vi "phan_upgrade13_2.vi"() -> ()   [LabVIEW 2019]
uses:
  <vilib>/Analysis/Matrix/Datatypes/RealMatrix.ctl
  <vilib>/Platform/TimedLoop/XDataNode/timing_clust.ctl
  <vilib>/Platform/TimedLoop/XDataNode/nitl_modes.ctl
  <vilib>/Platform/TimedLoop/XDataNode/wakeup.ctl
  <vilib>/imath/engines/lvmath2/RunTimeEngine/IndexRead/NIMS V(S).vi
  <instcachedir>/0/NIMS V(S)_0488751826AF41519A22953C041130DC.lvgen/NIMS V(S)_0488751826AF41519A22953C041130DC_000.vi
  <vilib>/imathl/engines/lvmath/Functions/Error Handling/Create Error.vi
  <vilib>/imath/engines/lvmath2/RunTimeEngine/NodeEndStatement/NIMS_NodeEndStatement_Output.vi
  <instcachedir>/0/NIMS_NodeEndStatement_Output_53EC0D466D134D7ABD903AC30B43404B.lvgen/NIMS_NodeEndStatement_Output_53EC0D466D134D7ABD903AC30B43404B_001.vi
  <vilib>/imath/engines/lvmath2/RunTimeEngine/ErrorHandling/NIMS_Finalize Error.vi
  <vilib>/imath/engines/lvmath2/RunTimeEngine/ArithmeticOperatorToken/NIMS_ArithmeticOperator_multmx(M,CV)-internal.vi
  <instcachedir>/0/NIMS_ArithmeticOperator_multmx(M,CV)-internal_2C55777844884EEDB828A940D397C7D0.lvgen/NIMS_ArithmeticOperator_multmx(M,CV)-internal_2C55777844884EEDB828A940D397C7D0_001.vi
  <vilib>/Analysis/Matrix/Numeric/Conversions/Matrix To Array - RM.vi
  <vilib>/imath/engines/lvmath2/RunTimeEngine/BuiltInFunctions/is_empty/NIMS_is_empty(GM).vi
  <instcachedir>/0/NIMS_is_empty(GM)_AF8F13F4B7FD436CB1855477E2504B8A.lvgen/NIMS_is_empty(GM)_AF8F13F4B7FD436CB1855477E2504B8A_004.vi
  <vilib>/imath/engines/lvmath2/RunTimeEngine/ArithmeticOperatorToken/NIMS_ArithmeticOperator_minus.vi
  <instcachedir>/0/NIMS_ArithmeticOperator_minus_12BFF9710EA5430A9EE87C5BC3F65186.lvgen/NIMS_ArithmeticOperator_minus_12BFF9710EA5430A9EE87C5BC3F65186_002.vi
  <vilib>/imath/engines/lvmath2/RunTimeEngine/ArithmeticOperatorToken/NIMS_ArithmeticOperator_plus.vi
  <instcachedir>/0/NIMS_ArithmeticOperator_plus_5C9385B0197D46E2B844C41E02F9EC39.lvgen/NIMS_ArithmeticOperator_plus_5C9385B0197D46E2B844C41E02F9EC39_003.vi
  <vilib>/imath/engines/lvmath2/RunTimeEngine/ErrorHandling/NIMS_Create Error From Enums.vi
  <vilib>/imath/engines/lvmath2/RunTimeEngine/RowToken/NIMS_RowToken_M_M.vi
  <instcachedir>/0/NIMS_RowToken_M_M_21FE36D058524603B8B587AC30FD72C2.lvgen/NIMS_RowToken_M_M_21FE36D058524603B8B587AC30FD72C2_004.vi
  <vilib>/imath/engines/lvmath2/RunTimeEngine/ArithmeticOperatorToken/NIMS_ArithmeticOperator_multmx(M,CV).vi
  <instcachedir>/0/NIMS_ArithmeticOperator_multmx(M,CV)_1D61EED49E1847F3B05DBB8EDD2FBF8F.lvgen/NIMS_ArithmeticOperator_multmx(M,CV)_1D61EED49E1847F3B05DBB8EDD2FBF8F_000.vi
  <vilib>/imath/engines/lvmath2/RunTimeEngine/IndexRead/NIMS M(S).vi
  <instcachedir>/0/NIMS M(S)_B826C018497E4940AE96BD27B540B6FB.lvgen/NIMS M(S)_B826C018497E4940AE96BD27B540B6FB_000.vi
  <vilib>/imath/engines/lvmath2/RunTimeEngine/BuiltInFunctions/abs/NIMS_abs(signed).vi
  <instcachedir>/0/NIMS_abs(signed)_C4FCB8E6058B49B797C7C8D53CA5F6EC.lvgen/NIMS_abs(signed)_C4FCB8E6058B49B797C7C8D53CA5F6EC_000.vi
  <vilib>/imath/engines/lvmath2/RunTimeEngine/VariableToken/NIMS_VariableToken_CondDefined.vi
  <instcachedir>/0/NIMS_VariableToken_CondDefined_30C3C94EAC01413DA882E848DEC89944.lvgen/NIMS_VariableToken_CondDefined_30C3C94EAC01413DA882E848DEC89944_003.vi
  <instcachedir>/0/NIMS_VariableToken_CondDefined_30C3C94EAC01413DA882E848DEC89944.lvgen/NIMS_VariableToken_CondDefined_30C3C94EAC01413DA882E848DEC89944_004.vi
  <instcachedir>/0/NIMS_VariableToken_CondDefined_30C3C94EAC01413DA882E848DEC89944.lvgen/NIMS_VariableToken_CondDefined_30C3C94EAC01413DA882E848DEC89944_001.vi
  <vilib>/Analysis/Matrix/Numeric/Conversions/Array To Matrix - RA2.vi
  <instcachedir>/0/NIMS_VariableToken_CondDefined_30C3C94EAC01413DA882E848DEC89944.lvgen/NIMS_VariableToken_CondDefined_30C3C94EAC01413DA882E848DEC89944_005.vi
  <vilib>/imath/engines/lvmath/Functions/Error Handling/MergeErrorsWrapper.vi
  <instcachedir>/0/NIMS_NodeEndStatement_Output_53EC0D466D134D7ABD903AC30B43404B.lvgen/NIMS_NodeEndStatement_Output_53EC0D466D134D7ABD903AC30B43404B_012.vi
  <instcachedir>/0/NIMS_NodeEndStatement_Output_53EC0D466D134D7ABD903AC30B43404B.lvgen/NIMS_NodeEndStatement_Output_53EC0D466D134D7ABD903AC30B43404B_010.vi
  <vilib>/platform/TimedLoop/XDataNode/XDataNode.xnode
  <vilib>/Platform/TimedLoop/XDataNode/XDNodeRunTimeDep.lvlib
  <vilib>/ptbypt/NI_PtbyPt.lvlib
  <vilib>/Analysis/Matrix/NI_Matrix.lvlib
panel:
  in  "yA":dbl
  in  "xA":dbl
  out "data out":string
  out "sosanh":dbl
  out "error out 2":errorcluster
  out "phi_k":dbl
  out "y_k":dbl
  out "x_k":dbl
  out "Real Matrix 2":T1
  out "Real Matrix":T1
  out "e_k":T1 caption="Real Matrix"
  out "error out":errorcluster
  out "y":dbl(graph)
  out "x":dbl(graph)
  out "y_1":dbl
  out "x_1":dbl
  out "y_0":dbl
  out "x_0":dbl
  out "wpre":dbl
  out "yo":dbl
  out "xo":dbl
  out "phi_ph":dbl
  out "wdk":dbl
  out "phi_sp":dbl
  in  "Kiw":dbl
  in  "Kpw":dbl=3.0
  in  "Kdw":dbl
  out "Vxdk":dbl
  out "Vydk":dbl
  out "Ts":dbl=10.0
  out "sailechvitri":cluster{"e_phi":dbl, "e_x":dbl, "e_y":dbl}(graph)
  in  "Kdxy":dbl
  in  "Kixy":dbl
  in  "Kpxy":dbl=4.0
  in  "?":T2(tab)
  out "time":dbl
  in  "phi_start":dbl=1.57 format="%#_13g"
  in  "phi_end":dbl=18.85
  in  "x0":dbl
  in  "w":dbl=0.2
  in  "y0":dbl
  in  "R":dbl=1.0
  in  "R":dbl=0.6
  in  "phi_end":dbl=18.85
  in  "phi_start":dbl format="%#_13g"
  in  "x0":dbl
  in  "w":dbl=0.5
  out "time 2":dbl
  in  "y0":dbl
  out "time":dbl
  in  "x":dbl
  in  "y":dbl
  in  "CONT":bool
  in  "vantoc":dbl=0.3
  in  "T":dbl
  out "time":dbl
  in  "camera update":bool
  out "xd":dbl
  out "yd":dbl
  out "phi":dbl
  out "time 3":dbl
  in  "phi_start 2":dbl format="%#_13g"
  in  "phi_end 2":dbl=31.4
  in  "x0 2":dbl
  in  "w 2":dbl=0.2
  in  "y0 2":dbl
  out "w_ph3":dbl
  out "w_ph2":dbl
  out "w_ph1":dbl
  in  "RESETMAP":bool=TRUE caption="Reset"
  out "duty3":dbl
  out "duty2":dbl
  out "duty1":dbl
  in  "RESET":bool
  out "Y_sp":dbl
  out "X_sp":dbl
  out "Y_ph":dbl
  out "X_ph":dbl
  out "Map":cluster{"Y":dbl[], "Y":dbl[]}[](graph)
  out "V3_sp":dbl
  out "V3_ph":dbl
  out "VAN TOC":T3(graph)
  in  "Kdv":dbl
  in  "Kiv":dbl=52.63
  in  "Kpv":dbl=1.337
  out "V2_ph":dbl
  out "V1_ph":dbl
  out "V2_sp":dbl
  out "V1_sp":dbl
  in  "START":bool
  # "HE THONG"
  # "PID VI TRI"
  # "PID TOC DO"
  # "VI TRI DIEU KHIEN\n(m)"
  # "VI TRI PHAN HOI\n(m)"
  # "Van toc dat"
  # "VAN TOC DIEU KHIEN\n(m/s)"
  # "VAN TOC PHAN HOI\n(m/s)"
  # "DUTY"
  # "TOC DO PHAN HOI (rad/s)"
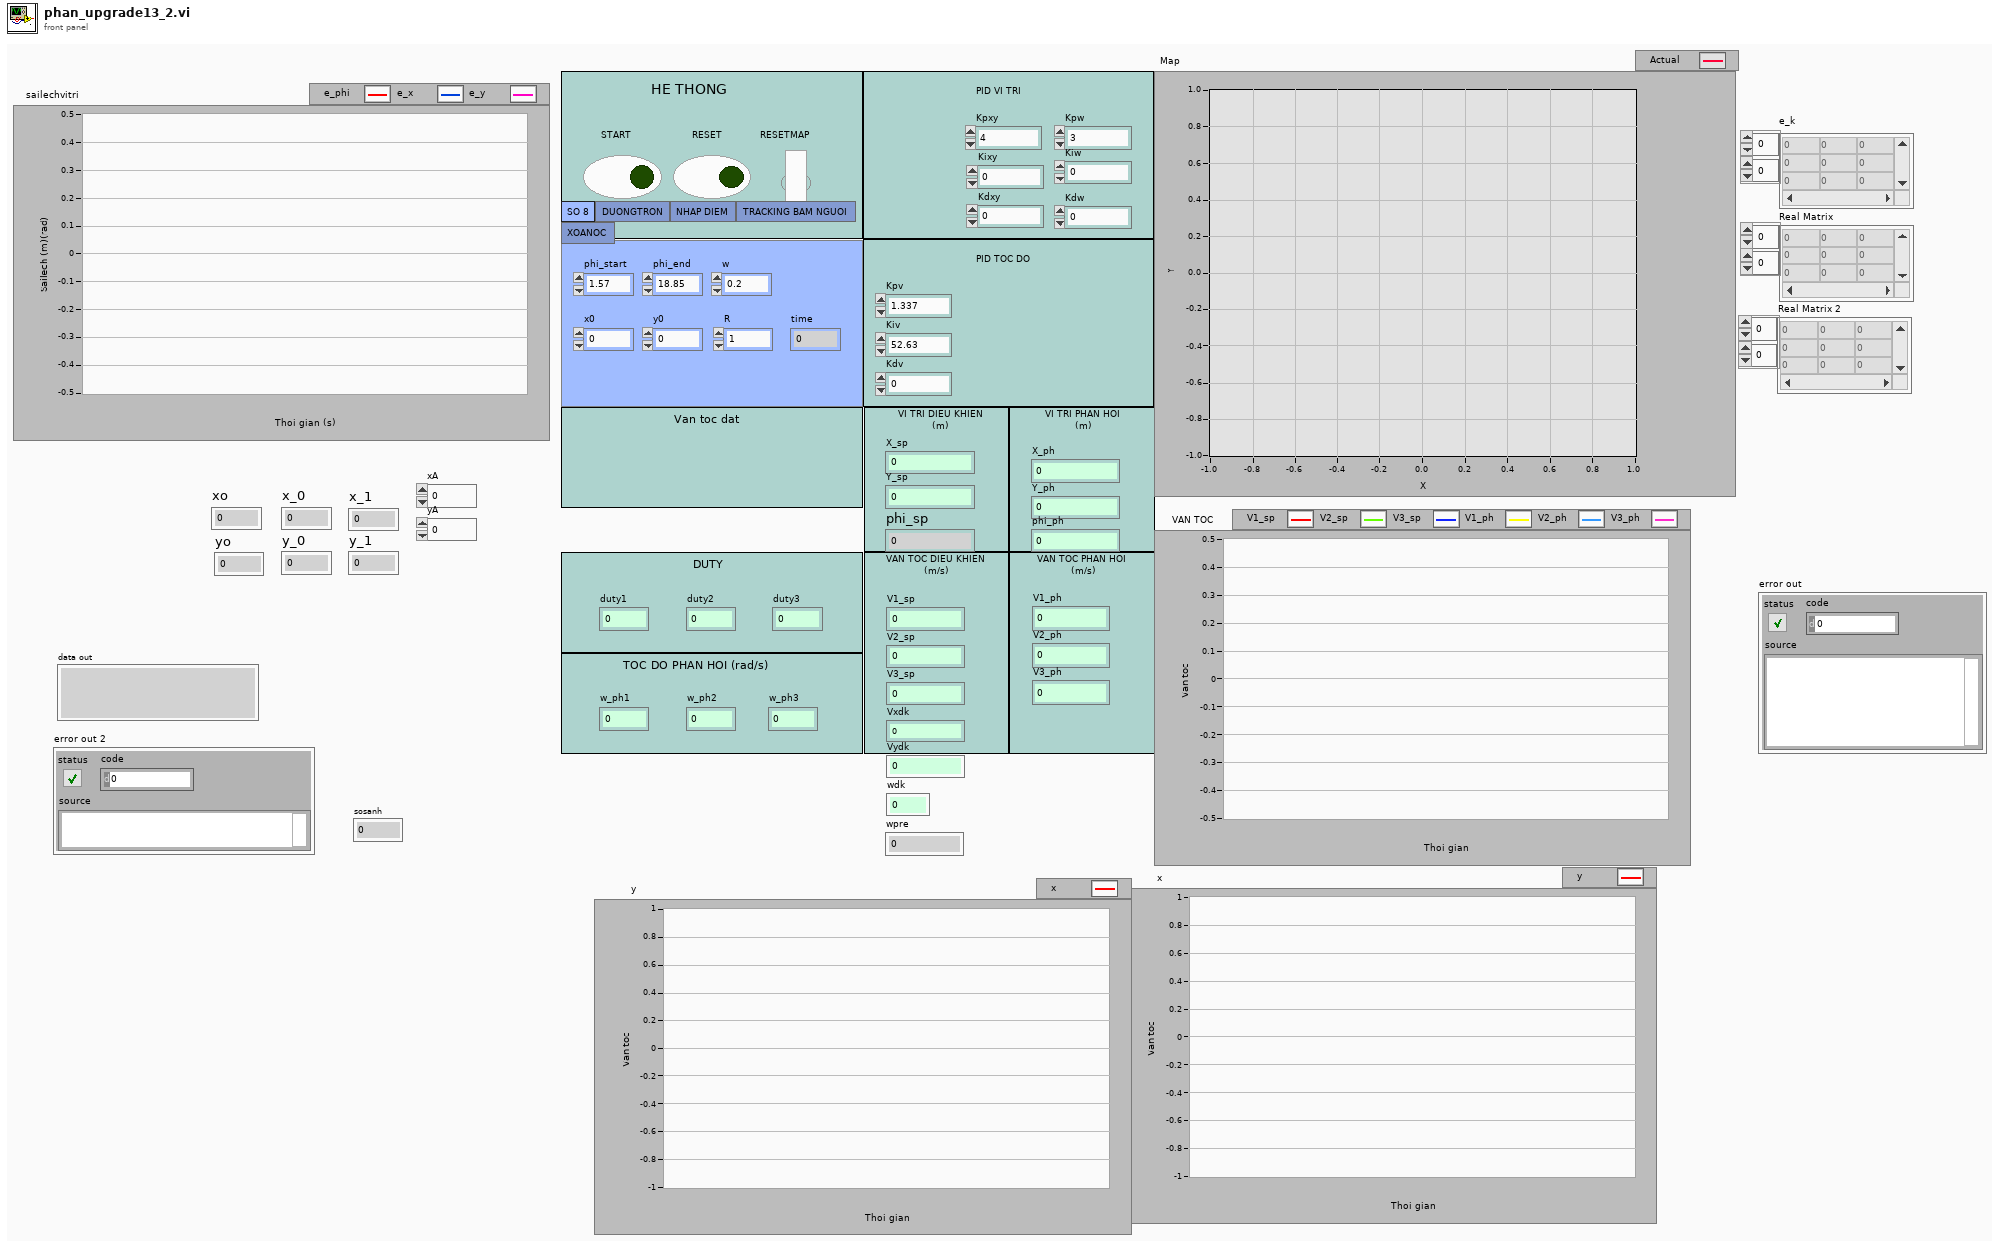
[diagram p1: front panel]
types:
  T1 = typedef "NI_Matrix.lvlib/RealMatrix.ctl" = dbl[][]
  T2 = enum32{"SO 8", "DUONGTRON", "NHAP DIEM", "TRACKING BAM NGUOI", "XOANOC"}
  T3 = cluster{dbl, dbl, "V1_ph":dbl, "V2_ph":dbl, dbl, "V3_ph":dbl}
  T4 = typedef "XDNodeRunTimeDep.lvlib/timing_clust.ctl" = cluster{"Expected End [f-1]":u64, "Actual End [f-1]":u64, "Finished Late? [f-1]":bool, "Expected End [i-1]":u64, "Actual End [i-1]":u64, "Finished Late? [i-1]":bool, "Expected Start [i]":u64, "Actual Start [i]":u64, "Expected Start [f]":u64, "Actual Start [f]":u64, "Source Name":string, "Structure Name":string, "Period":i64, "Deadline":i64, "Offset":i64, "Start":i64, "Priority":i32, "Timeout":i32, "Mode":T5, "Wakeup Reason":T6, "Error":errorcluster, "Source Type":string, "Secondary Source Type":string, "Global End Time":u64, "Global Start Time":u64, "Frame Duration":u64, "Iteration Duration":u64, "Assigned CPU":i32, "I/O Scan Engine Mode":u32}
  T5 = typedef "XDNodeRunTimeDep.lvlib/nitl_modes.ctl" = enum32{"No Change", "Process missed periods, maintain original phase", "Discard missed periods, maintain original phase", "Process missed periods, ignore original phase", "Discard missed periods, ignore original phase"}
  T6 = typedef "XDNodeRunTimeDep.lvlib/wakeup.ctl" = enum32{"Normal", "Aborted", "Asynchronous wakeup", "Timing source error", "Timed loop error", "Timeout"}
  T7 = enum16{"Standard", "Buffered", "CRLF", "Immediate"}
  T8 = cluster{"V1_sp":dbl, "V2_sp":dbl, "V3_sp":dbl, "V_ph1":dbl, "V_ph2":dbl, "V_ph3":dbl}
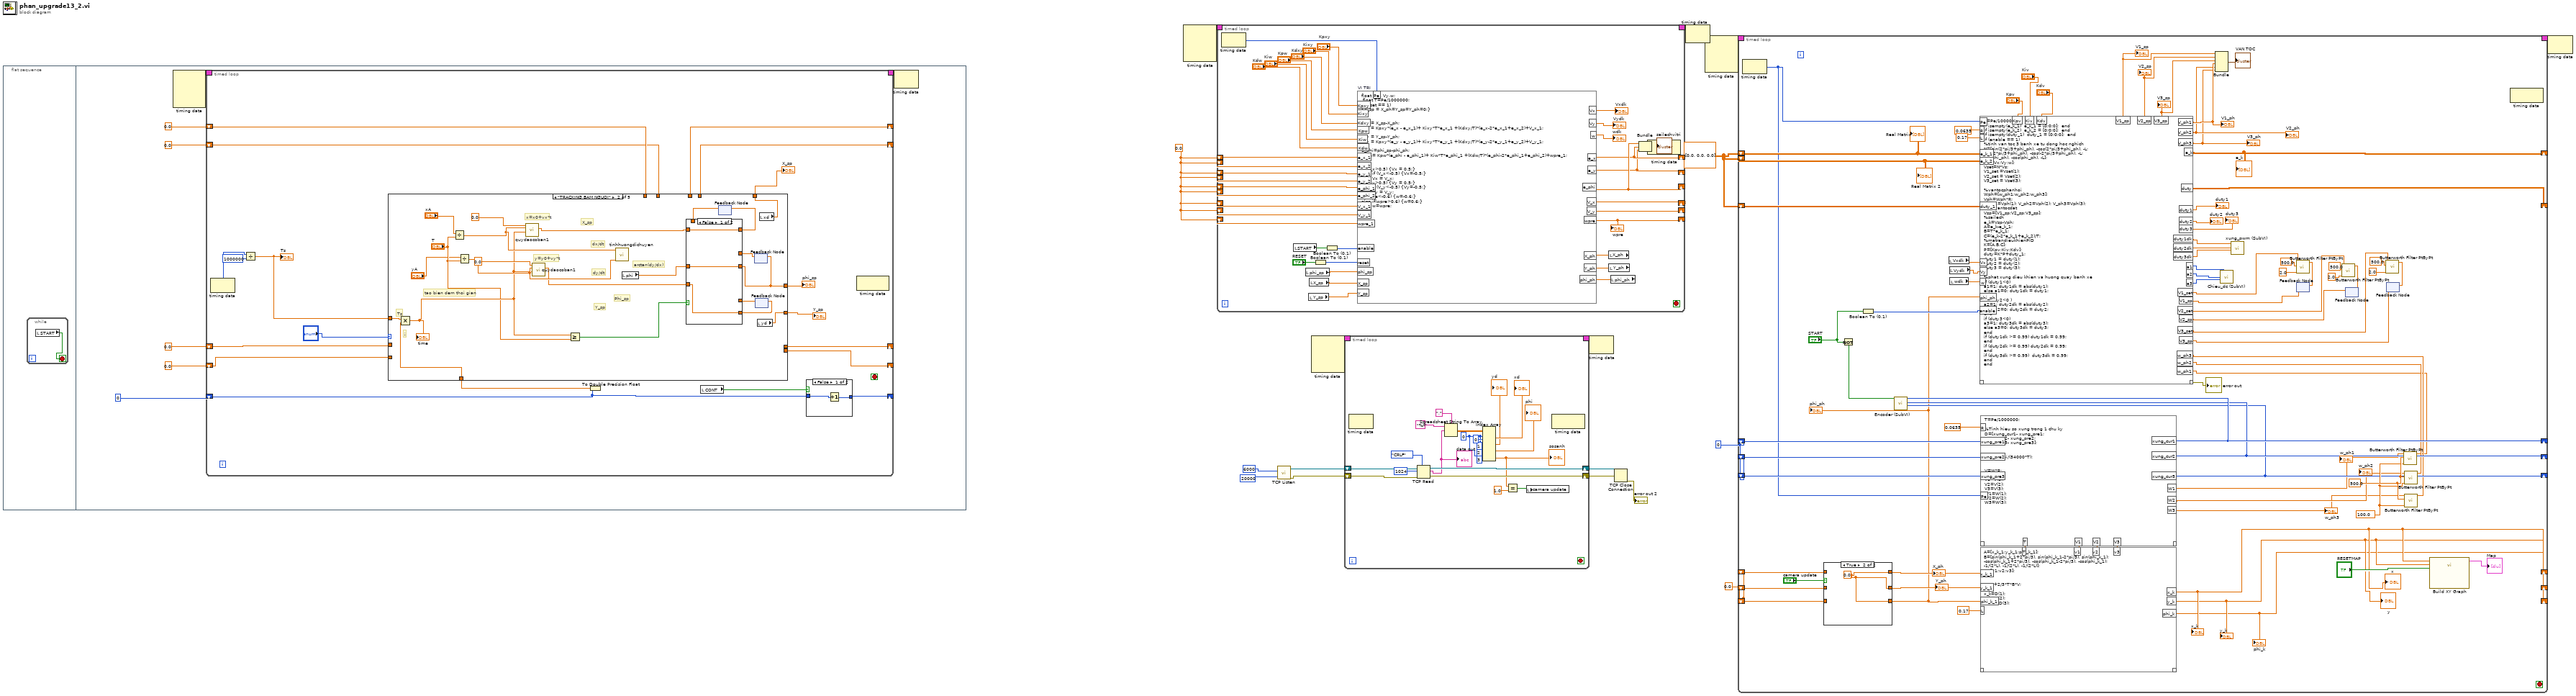
[diagram p0: block diagram]
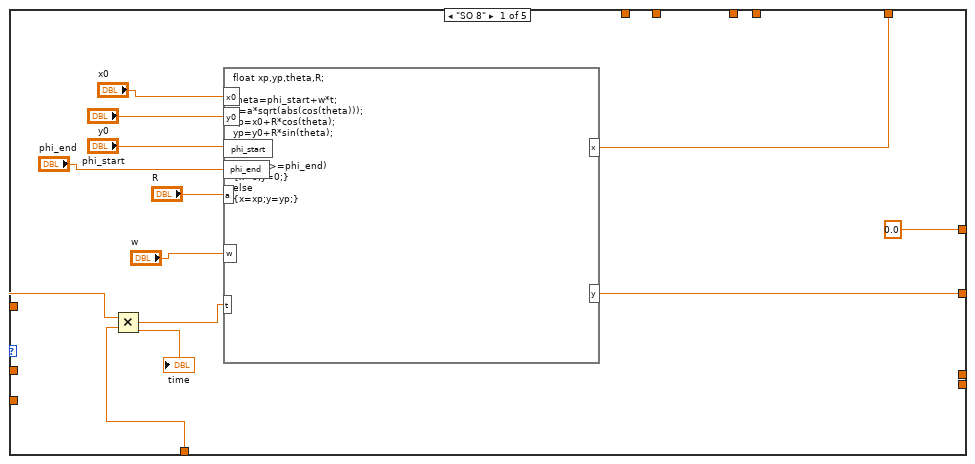
[diagram p2: hidden frame]
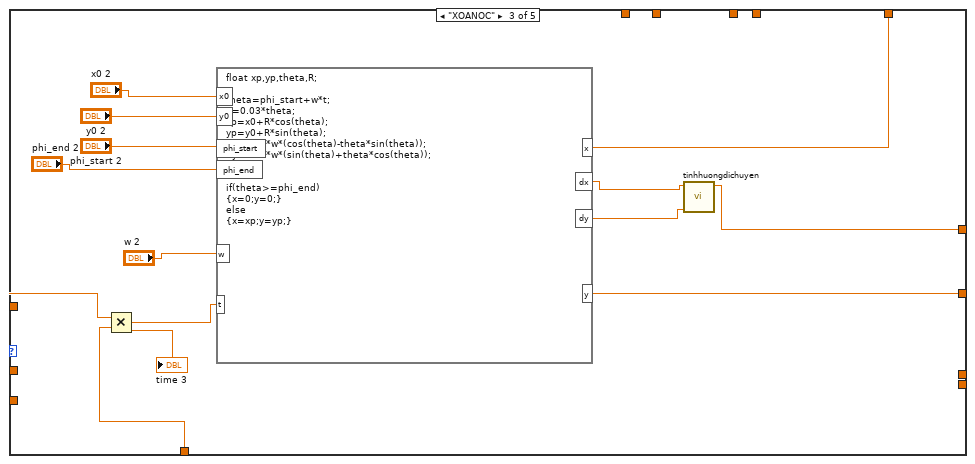
[diagram p4: hidden frame]
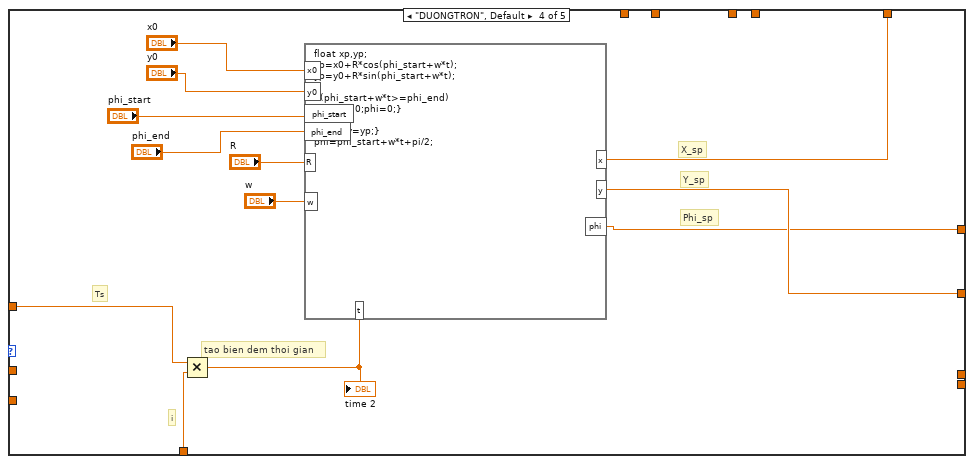
[diagram p5: hidden frame]
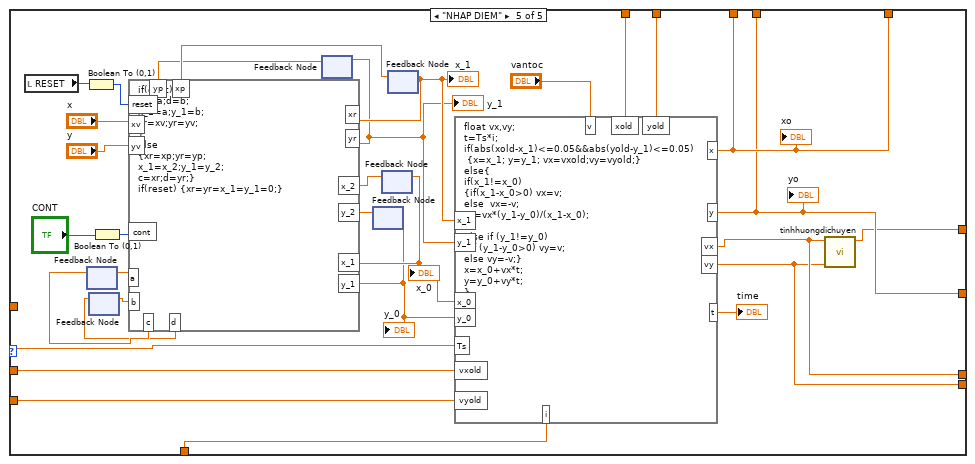
[diagram p6: hidden frame]
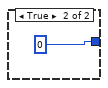
[diagram p7: hidden frame]
diagram:
  w11 = T1 [[0.0], [0.0], [0.0]] ("Real Matrix")
  w12 = 0 ("Counter Value")
  w13 = 0.0 ("e_x")
  w10 = 0.0 ("e1")
  n1 = flat-sequence {
    frame #0 {
      n2 = while {
        stop <- w18 stop-if-true
        n3 = local read "START"() -> (w18:bool)
      }
    }
    frame #1 {
      n4 = node-c288() -> (w25:T4)  [unwired: 4 in]
      n5 = timed-loop {
        timing: w25 -> [_]
        timing-out: [_] -> w24
        shift-right: [w43] -> _
        shift-left: 0 -> [w42]
        shift-right: [w34] -> _
        shift-left: 0.0 -> [w32]
        shift-right: [w33] -> _
        shift-left: 0.0 -> [w31]
        shift-right: [w30] -> _
        shift-left: 0.0 ("x") -> [w28]
        shift-right: [w29] -> _
        shift-left: 0.0 ("y") -> [w27]
        stop <- _ stop-if-true
        n6 = node-c288() -> (w41:i64)  [unwired: 1 in]
        n7 = Divide(x=w41, y=i64 1000000) -> (x/y=w39:dbl)
        "Ts" <- w39
        n8 = To Double Precision Float(number=w42) -> (double precision float=w44:dbl)
        n9 = case shown="\"TRACKING BAM NGUOI\"" "?" {
          tunnel: w44 -> [w55 w78 w90 w108 w140]
          tunnel: [w47 w58 w88 w100 w114] -> w38
          tunnel: [w46 w57 w89 w99 w113] -> w37
          tunnel: [0.0 ("phi_0") w65 w85 w98 w110] -> w36
          tunnel: w39 -> [w56 w77 w91 w109 w120]
          tunnel: [_ _ _ _ w118] -> w34
          tunnel: [_ _ _ _ w117] -> w33
          tunnel: w32 -> [_ _ _ _ w116]
          tunnel: w31 -> [_ _ _ _ w115]
          tunnel: [_ _ _ _ w114] -> w30
          tunnel: [_ _ _ _ w113] -> w29
          tunnel: w28 -> [_ _ _ _ w112]
          tunnel: w27 -> [_ _ _ _ w111]
          frame "SO 8" {
            n10 = Multiply(x=w56, y=w55) -> (x*y=w54:dbl)
            "time" <- w54
            n11 = formula code="float xp,yp,theta,R;\n\ntheta=phi_start+w*t;\nR=a*sqrt(abs(cos(theta)));\nxp=x0+R*cos(theta);\nyp=y0+R*sin(theta);\n\n\nif(theta>=phi_end)\n{x=0;y=0;}\nelse\n{x=xp;y=yp;}"("t"=w54, "w"="w", "x0"="x0", "y0"="y0", "phi_start"="phi_start", "phi_end"="phi_end", "a"="R") -> ("x"=w47:dbl, "y"=w46:dbl)
          }
          frame "TRACKING BAM NGUOI" {
            # "Y_sp"
            # "Phi_sp"
            # "X_sp"
            # "arctan(dy/dx)"
            # "dy/dt"
            # "dx/dt"
            # "Ts"
            # "i"
            # "y=y0+vy*t"
            # "x=x0+vx*t"
            # "tao bien dem thoi gian"
            n12 = Multiply(x=w77, y=w78) -> (x*y=w72:dbl)
            "time" <- w72
            n13 = Divide(x="xA", y="T") -> (x/y=w74:dbl)
            n14 = Divide(x="yA", y="T") -> (x/y=w73:dbl)
            n15 = call "quydaocoban1.vi"("t"=w72, "v"=w74, "S0"=0.0 ("x0")) -> ("S"=w69:dbl)  [unwired: 8 in]
            n16 = call "quydaocoban1.vi"("t"=w72, "v"=w73, "S0"=0.0 ("y0")) -> ("S"=w68:dbl)  [unwired: 8 in]
            n17 = Greater Or Equal?(x=w72, y="T") -> (x >= y?=w70:bool)
            n18 = call "tinhhuongdichuyen.vi"("dy"=w73, "dx"=w74) -> ()  [unwired: 9 in, 1 out]
            n19 = local read "phi"() -> (w61:dbl)
            n20 = feedback #1() -> (w66:dbl)  [unwired: 1 in]
            n21 = feedback #2() -> (w64:dbl)  [unwired: 1 in]
            n22 = feedback #3() -> (w62:dbl)  [unwired: 1 in]
            n23 = case shown="False" w70 {
              tunnel: w69 -> [w81 _]
              tunnel: [w81 w84] -> w67
              tunnel: w61 -> [w80 _]
              tunnel: [w80 w83] -> w65
              tunnel: w68 -> [w79 _]
              tunnel: [w79 w82] -> w63
              tunnel: w66 -> [_ w84]
              tunnel: w64 -> [_ w83]
              tunnel: w62 -> [_ w82]
              frame False {
              }
              frame True {
              }
            }
            n24 = feedback-in #1(w67) -> ()
            n25 = feedback-in #2(w65) -> ()
            n26 = feedback-in #3(w63) -> ()
            n27 = local read "yd"() -> (w57:dbl)
            n28 = local read "xd"() -> (w58:dbl)
          }
          frame "XOANOC" {
            n29 = Multiply(x=w91, y=w90) -> (x*y=w97:dbl)
            "time 3" <- w97
            n30 = formula code="float xp,yp,theta,R;\n\ntheta=phi_start+w*t;\nR=0.03*theta;\nxp=x0+R*cos(theta);\nyp=y0+R*sin(theta);\ndx=0.03*w*(cos(theta)-theta*sin(theta));\ndy=0.03*w*(sin(theta)+theta*cos(theta));\n\n\nif(theta>=phi_end)\n{x=0;y=0;}\nelse\n{x=xp;y=yp;}"("t"=w97, "w"="w 2", "x0"="x0 2", "y0"="y0 2", "phi_start"="phi_start 2", "phi_end"="phi_end 2") -> ("x"=w88:dbl, "y"=w89:dbl, "dx"=w87:dbl, "dy"=w86:dbl)
            n31 = call "tinhhuongdichuyen.vi"("dy"=w86, "dx"=w87) -> ("phi"=w85:dbl)  [unwired: 9 in]
          }
          frame "DUONGTRON", Default {
            # "Phi_sp"
            # "Y_sp"
            # "X_sp"
            # "i"
            # "Ts"
            # "tao bien dem thoi gian"
            n32 = Multiply(x=w109, y=w108) -> (x*y=w107:dbl)
            "time 2" <- w107
            n33 = formula code="float xp,yp;\nxp=x0+R*cos(phi_start+w*t);\nyp=y0+R*sin(phi_start+w*t);\n\nif(phi_start+w*t>=phi_end)\n{x=0;y=0;phi=0;}\nelse\n{x=xp;y=yp;}\nphi=phi_start+w*t+pi/2;"("t"=w107, "w"="w", "x0"="x0", "y0"="y0", "phi_start"="phi_start", "phi_end"="phi_end", "R"="R") -> ("x"=w100:dbl, "y"=w99:dbl, "phi"=w98:dbl)
          }
          frame "NHAP DIEM" {
            n34 = local read "RESET"() -> (w122:bool)
            n35 = Boolean To (0,1)(Boolean=w122) -> (0, 1=w121:i16)
            n36 = feedback #4() -> (w125:dbl)  [unwired: 1 in]
            n37 = feedback #5() -> (w123:dbl)  [unwired: 1 in]
            n38 = Boolean To (0,1)(Boolean="CONT") -> (0, 1=w137:i16)
            n39 = feedback #6() -> (w131:dbl)  [unwired: 1 in]
            n40 = feedback #7() -> (w128:dbl)  [unwired: 1 in]
            n41 = feedback #8() -> (w130:dbl)  [unwired: 1 in]
            n42 = feedback #9() -> (w132:dbl)  [unwired: 1 in]
            n43 = formula code="if(cont)\n{c=a;d=b;\nx_1=a;y_1=b;\nxr=xv;yr=yv;\n}\nelse \n{xr=xp;yr=yp;\nx_1=x_2;y_1=y_2;\nc=xr;d=yr;}\nif(reset) {xr=yr=x_1=y_1=0;}"("cont"=w137, "xv"="x", "yv"="y", "yp"=w131, "xp"=w132, "x_2"=w130, "y_2"=w128, "a"=w125, "b"=w123, "reset"=w121) -> ("xr"=w134:dbl, "yr"=w133:dbl, "x_1"=w129:dbl, "y_1"=w127:dbl, "c"=w126:dbl, "d"=w124:dbl)
            "x_0" <- w129
            "y_0" <- w127
            "x_1" <- w134
            "y_1" <- w133
            n44 = feedback-in #4(w126) -> ()
            n45 = feedback-in #5(w124) -> ()
            n46 = feedback-in #6(w133) -> ()
            n47 = feedback-in #7(w127) -> ()
            n48 = feedback-in #8(w129) -> ()
            n49 = feedback-in #9(w134) -> ()
            n50 = formula code="float vx,vy;\nt=Ts*i;\nif(abs(xold-x_1)<=0.05&&abs(yold-y_1)<=0.05)\n {x=x_1; y=y_1; vx=vxold;vy=vyold;}\nelse{\nif(x_1!=x_0)\n{if(x_1-x_0>0) vx=v;\nelse  vx=-v;\nvy=vx*(y_1-y_0)/(x_1-x_0);\n}\nelse if (y_1!=y_0) \n{if (y_1-y_0>0) vy=v;\nelse vy=-v;}\nx=x_0+vx*t;\ny=y_0+vy*t;\n}"("i"=w140, "x_1"=w134, "y_1"=w133, "x_0"=w129, "y_0"=w127, "Ts"=w120, "v"="vantoc", "xold"=w112, "yold"=w111, "vxold"=w116, "vyold"=w115) -> ("x"=w114:dbl, "y"=w113:dbl, "vx"=w118:dbl, "t"=→"time":dbl, "vy"=w117:dbl)
            "xo" <- w114
            "yo" <- w113
            n51 = call "tinhhuongdichuyen.vi"("dy"=w117, "dx"=w118) -> ("phi"=w110:dbl)  [unwired: 9 in]
          }
        }
        "X_sp" <- w38
        "Y_sp" <- w37
        "phi_sp" <- w36
        n52 = local read "CONT"() -> (w26:bool)
        n53 = case shown="False" w26 {
          tunnel: [w142 0] -> w43
          tunnel: w42 -> [w141 _]
          frame False {
            n54 = Increment(x=w141) -> (x+1=w142:i32)
          }
          frame True {
          }
        }
        n55 = node-c288() -> ()  [unwired: 1 in, 1 out]
      }
      n56 = node-c288(w24) -> ()  [unwired: 1 out]
    }
  }
  n57 = node-c288() -> (w15:T4)  [unwired: 4 in]
  n58 = timed-loop {
    timing: w15 -> [_]
    timing-out: [_] -> w14
    shift-right: [w169] -> _
    shift-left: w13 -> [w177]
    shift-left: w13 -> [w176]
    shift-right: [w152] -> _
    shift-left: w13 -> [w175]
    shift-left: w13 -> [w174]
    shift-right: [w170] -> _
    shift-left: w13 -> [w173]
    shift-left: w13 -> [w172]
    shift-right: [w157] -> _
    shift-left: w13 -> [w160]
    shift-right: [w156] -> _
    shift-left: w13 -> [w159]
    shift-right: [w155] -> _
    shift-left: w13 -> [w158]
    stop <- _ stop-if-true
    # "Gioihantocdo"
    # "BodieukhienPIDvitri"
    n59 = node-c288() -> (w184:i64)  [unwired: 1 in]
    n60 = local read "START"() -> (w154:bool)
    n61 = local read "phi_sp"() -> (w150:dbl)
    n62 = local read "Y_sp"() -> (w149:dbl)
    n63 = local read "X_sp"() -> (w151:dbl)
    n64 = Boolean To (0,1)(Boolean="RESET") -> (0, 1=w167:i16)
    n65 = Boolean To (0,1)(Boolean=w154) -> (0, 1=w153:i16)
    n66 = local read "X_ph"() -> (w166:dbl)
    n67 = local read "Y_ph"() -> (w165:dbl)
    n68 = local read "phi_ph"() -> (w164:dbl)
    n69 = formula code="float  Vx, Vy,w;\n float T=Pe/1000000;\nif(reset == 1)\n{X_sp = X_ph=Y_sp=Y_ph=0;}\n \n\ne_x = X_sp-X_ph; \nV_x = Kpxy*(e_x - e_x_1)+ Kixy*T*e_x_1 +(Kdxy/T)*(e_x-2*e_x_1+e_x_2)+V_x_1;\n\ne_y = Y_sp-Y_ph; \nV_y = Kpxy*(e_y - e_y_1)+ Kixy*T*e_y_1 +(Kdxy/T)*(e_y-2*e_y_1+e_y_2)+V_y_1;\n\ne_phi=phi_sp-phi_ph;\nwpre= Kpw*(e_phi - e_phi_1)+ Kiw*T*e_phi_1 +(Kdw/T)*(e_phi-2*e_phi_1+e_phi_2)+wpre_1;\n\n\nif (V_x>0.5) {Vx = 0.5;} \nelse if (V_x<-0.5) {Vx=-0.5;}\nelse Vx = V_x;\nif (V_y>0.5) {Vy = 0.5;} \nelse if (V_y<-0.5) {Vy=-0.5;}\nelse Vy = V_y;\nif (wpre<-0.6) {w=-0.6;}\nelse if(wpre>0.6) {w=0.6;}\nelse w=wpre;" "VI TRI"("Kpxy"="Kpxy", "Kixy"="Kixy", "Kdxy"="Kdxy", "Kpw"="Kpw", "Kiw"="Kiw", "Kdw"="Kdw", "Pe"=w184, "e_x_1"=w177, "e_x_2"=w176, "e_y_1"=w175, "e_y_2"=w174, "e_phi_1"=w173, "e_phi_2"=w172, "reset"=w167, "phi_sp"=w150, "X_sp"=w151, "Y_sp"=w149, "X_ph"=w166, "Y_ph"=w165, "phi_ph"=w164, "V_x_1"=w160, "V_y_1"=w159, "wpre_1"=w158, "enable"=w153) -> ("e_x"=w169:dbl, "e_y"=w152:dbl, "e_phi"=w170:dbl, "Vx"=→"Vxdk":dbl, "Vy"=→"Vydk":dbl, "w"=→"wdk":dbl, "V_x"=w157:dbl, "V_y"=w156:dbl, "wpre"=w155:dbl)
    "wpre" <- w155
    n70 = Bundle("e_phi"=w170, "e_x"=w169, "e_y"=w152) -> (→"sailechvitri":cluster{"e_phi":dbl, "e_x":dbl, "e_y":dbl})  [unwired: 1 in]
    n71 = node-c288() -> ()  [unwired: 1 in, 1 out]
  }
  n72 = call <vilib>:"TCP Listen.vi"("timeout ms (wait forever: -1)"=20000, "port"=u16 6000) -> ("error out"=w4:errorcluster, "connection ID"=w3:refnum<k5>)  [unwired: 5 in, 3 out]
  n73 = node-c288() -> (w9:T4)  [unwired: 4 in]
  n74 = timed-loop {
    timing: w9 -> [_]
    timing-out: [_] -> w8
    shift-right: [w206] -> w2
    shift-left: w4 -> [w208]
    shift-right: [w205] -> w1
    shift-left: w3 -> [w207]
    stop <- _ stop-if-true
    w192 = 0 ("index (row)")
    n75 = node-c288() -> ()  [unwired: 1 in, 1 out]
    n76 = TCP Read(connection ID=w207, bytes to read=1024, error in (no error)=w208, 7:T7."CRLF" ("mode (standard)")) -> (connection ID out=w205:refnum<k5>, data out=w204:string, error out=w206:errorcluster)  [unwired: 1 in]
    "data out" <- w204
    n77 = Spreadsheet String To Array(delimiter (Tab)=",", format string="%f", spreadsheet string=w204) -> (array=w200:dbl[][])  [unwired: 1 in]
    n78 = Index Array(array=w200, index (row) #1=w192, index (col) #1=0 ("disabled index (col)"), index (row) #2=w192, index (col) #2=1 ("disabled index (col)"), index (row) #3=w192, index (col) #3=2 ("disabled index (col)"), index (row) #4=w192, index (col) #4=3 ("disabled index (col)")) -> (element #1=→"xd":dbl, element #2=→"yd":dbl, element #3=→"phi":dbl, element #4=w189:dbl)
    "sosanh" <- w189
    n79 = Equal?(x=w189, y=1.0) -> (x = y?=w188:bool)
    n80 = local write "camera update"(w188) -> ()
    n81 = node-c288() -> ()  [unwired: 1 in, 1 out]
  }
  n82 = node-c288(w8) -> ()  [unwired: 1 out]
  n83 = TCP Close Connection(connection ID=w1, error in (no error)=w2) -> (error out=→"error out 2":errorcluster)  [unwired: 1 in, 1 out]
  n84 = node-c288(w14) -> ()  [unwired: 1 out]
  n85 = node-c288() -> (w17:T4)  [unwired: 4 in]
  n86 = timed-loop {
    timing: w17 -> [_]
    timing-out: [_] -> w16
    shift-right: [w248] -> _
    shift-left: w11 -> [w229]
    shift-right: [w274] -> _
    shift-left: w10 -> [w217]
    shift-right: [w273] -> _
    shift-left: w10 -> [w215]
    shift-right: [w267] -> _
    shift-left: w12 -> [w270]
    shift-right: [w266] -> _
    shift-left: w12 -> [w269]
    shift-right: [w265] -> _
    shift-left: w12 -> [w268]
    shift-left: w11 -> [w228]
    shift-right: [w272] -> _
    shift-left: w10 -> [w213]
    shift-right: [w221] -> _
    shift-left: w11 -> [w222]
    stop <- _ stop-if-true
    w287 = 100.0 ("flw")
    w288 = 500.0 ("sampling freq: fs")
    # "Tinh van toc"
    # "Tinh toc do goc"
    # "Tinh vi tri phan hoi tu van toc qua dong hoc thuan"
    n87 = node-c288() -> (w220:i64)  [unwired: 1 in]
    n88 = case shown="True" "camera update" {
      tunnel: w217 -> [w294 _]
      tunnel: [w294 w295] -> w216
      tunnel: w215 -> [w293 _]
      tunnel: [w293 w295] -> w214
      tunnel: w213 -> [w292 _]
      tunnel: [w292 w295] -> w212
      frame False {
      }
      frame True {
        w295 = 0.0
      }
    }
    "X_ph" <- w216
    "Y_ph" <- w214
    "phi_ph" <- w212
    n89 = Not(x="START") -> (.not. x?=w289:bool)
    n90 = Boolean To (0,1)(Boolean="START") -> (0, 1=w219:i16)
    n91 = call "Encoder (SubVI).vi"("Boolean"=w289) -> ("Counter Value3"=w265:i32, "Counter Value 2"=w266:i32, "Counter Value"=w267:i32)  [unwired: 8 in]
    n92 = local read "Vxdk"() -> (w227:dbl)
    n93 = local read "Vydk"() -> (w226:dbl)
    n94 = local read "wdk"() -> (w225:dbl)
    n95 = mathscript code="T=Pe/1000000;\n\n%Tinh hieu so xung trong 1 chu ky\nD=[xung_cur1- xung_pre1;\nxung_cur2- xung_pre2;\nxung_cur3- xung_pre3];\n\n\nW=D*2*pi/(54000*T);\n\n\nV=W*R;\n\nV1=V(1);\nV2=V(2);\nV3=V(3);\nW1=W(1);\nW2=W(2);\nW3=W(3);"("xung_pre1"=w270, "xung_pre2"=w269, "xung_pre3"=w268, "xung_cur1"=w267, "xung_cur2"=w266, "xung_cur3"=w265, "R"=0.0635 ("input variable"), "Pe"=w220) -> ("W1"=w264:dbl, "W2"=w263:dbl, "W3"=w262:dbl, "T"=w261:dbl, "V1"=w260:dbl, "V2"=w259:dbl, "V3"=w258:dbl)  [unwired: 1 in, 1 out]
    "w_ph1" <- w264
    "w_ph2" <- w263
    "w_ph3" <- w262
    n96 = mathscript code="A=[x_k_1;y_k_1;phi_k_1];\nB=[sin(phi_k_1+2*pi/3), sin(phi_k_1-2*pi/3), sin(phi_k_1);\n-cos(phi_k_1+2*pi/3), -cos(phi_k_1-2*pi/3), -cos(phi_k_1);\n-1/(2*L), -1/(2*L), -1/(2*L)];\nV=[v1;v2;v3];\n\n\nD=A+2/3*T*B*V;\n\nx_k=D(1);\ny_k=D(2);\nphi_k=D(3);"("x_k_1"=w216, "y_k_1"=w214, "phi_k_1"=w212, "T"=w261, "v1"=w260, "v2"=w259, "v3"=w258, "L"=0.17) -> ("x_k"=w274:dbl, "y_k"=w273:dbl, "phi_k"=w272:dbl)  [unwired: 1 in, 1 out]
    "x" <- w274
    "y" <- w273
    "x_k" <- w274
    "y_k" <- w273
    "phi_k" <- w272
    n97 = feedback #10() -> (w239:dbl)  [unwired: 1 in]
    n98 = feedback #11() -> (w237:dbl)  [unwired: 1 in]
    n99 = feedback #12() -> (w235:dbl)  [unwired: 1 in]
    n100 = call <vilib>:"Butterworth Filter PtByPt.vi"("low cutoff freq: fl"=w287, "sampling freq: fs"=w288, "x"=w264) -> ("Filtered x"=w232:dbl)  [unwired: 6 in, 1 out]
    n101 = call <vilib>:"Butterworth Filter PtByPt.vi"("low cutoff freq: fl"=w287, "sampling freq: fs"=w288, "x"=w263) -> ("Filtered x"=w233:dbl)  [unwired: 6 in, 1 out]
    n102 = call <vilib>:"Butterworth Filter PtByPt.vi"("low cutoff freq: fl"=w287, "sampling freq: fs"=w288, "x"=w262) -> ("Filtered x"=w234:dbl)  [unwired: 6 in, 1 out]
    n103 = mathscript code="T=Pe/1000000;\nif isempty(e_k_1)  e_k_1 = [0;0;0];  end\nif isempty(e_k_2)  e_k_2 = [0;0;0];  end\nif isempty(duty_1)  duty_1 = [0;0;0];  end\nif (enable == 1)\n%tinh van toc 3 banh xe tu dong hoc nghich\nN=[sin(2*pi/3+phi_ph), -cos(2*pi/3+phi_ph), -L;\nsin(-2*pi/3+phi_ph), -cos(-2*pi/3+phi_ph), -L;\nsin(phi_ph), -cos(phi_ph), -L];\nVs=[Vx;Vy;w];\nVset=N*Vs;\nV1_set =Vset(1);\nV2_set = Vset(2);\nV3_set = Vset(3);\n\n%vantocphanhoi\nWph=[w_ph1;w_ph2;w_ph3];\nVph=Wph*R;\nV_ph1=Vph(1); V_ph2=Vph(2); V_ph3=Vph(3);\n%locvantocdat\nVsp=[V1_sp;V2_sp;V3_sp];\n%sailech\ne_k=Vsp-Vph;\nA=e_k-e_k_1;\nB=T*e_k_1;\nC=(e_k-2*e_k_1+e_k_2)/T;\n%matrandieukhienPID\nK=[A,B,C];\nP=[Kpv;Kiv;Kdv];\nduty=K*P+duty_1;\nduty1 = duty(1);\nduty2 = duty(2);\nduty3 = duty(3);\n\n%phat xung dieu khien va huong quay banh xe\nif (duty1<0)  \na1=1; duty1dk = abs(duty1);\nelse a1=0; duty1dk = duty1;\nend\nif (duty2<0 ) \na2=1; duty2dk = abs(duty2);\nelse a2=0; duty2dk = duty2;\nend\nif (duty3<0)  \na3=1; duty3dk = abs(duty3);\nelse a3=0; duty3dk = duty3;\nend \nif (duty1dk >= 0.99) duty1dk = 0.99;\nend\nif (duty2dk >= 0.99) duty2dk = 0.99;\nend\nif (duty3dk >= 0.99)  duty3dk = 0.99;\nend\nend"("Pe"=w220, "Kpv"="Kpv", "Kiv"="Kiv", "Kdv"="Kdv", "phi_ph"=w212, "enable"=w219, "R"=0.0635 ("input variable"), "L"=0.17 ("input variable"), "e_k_1"=w229, "e_k_2"=w228, "Vx"=w227, "Vy"=w226, "w"=w225, "V1_sp"=w239, "V2_sp"=w237, "V3_sp"=w235, "w_ph3"=w234, "w_ph2"=w233, "w_ph1"=w232, "duty_1"=w222) -> ("??"=→"error out":errorcluster, "V1_sp"=w254:dbl, "V2_sp"=w253:dbl, "V3_sp"=w252:dbl, "V_ph1"=w251:dbl, "V_ph2"=w250:dbl, "V_ph3"=w249:dbl, "e_k"=w248:T1, "duty1"=→"duty1":dbl, "duty2"=→"duty2":dbl, "duty3"=→"duty3":dbl, "duty1dk"=w246:dbl, "duty2dk"=w245:dbl, "duty3dk"=w244:dbl, "a1"=w243:i32, "a2"=w242:i32, "a3"=w241:i32, "V1_set"=w240:dbl, "V2_set"=w238:dbl, "V3_set"=w236:dbl, "duty"=w221:T1)  [unwired: 1 in]
    "V1_sp" <- w254
    "V2_sp" <- w253
    "V1_ph" <- w251
    "V2_ph" <- w250
    "V3_ph" <- w249
    "V3_sp" <- w252
    "e_k" <- w248
    n104 = Bundle("V1_sp"=w254, "V2_sp"=w253, "V3_sp"=w252, "V_ph1"=w251, "V_ph2"=w250, "V_ph3"=w249) -> (→"VAN TOC":T8)  [unwired: 1 in]
    n105 = call "Chieu_dc (SubVI).vi"("a3"=w241, "a2"=w242, "a1"=w243) -> ()
    n106 = call "xung_pwm (SubVI).vi"("duty3 in"=w244, "duty2 in"=w245, "duty1 in"=w246) -> ()  [unwired: 6 in, 3 out]
    n107 = call <vilib>:"Butterworth Filter PtByPt.vi"("low cutoff freq: fl"=2.0, "sampling freq: fs"=500.0, "x"=w240) -> ("Filtered x"=w280:dbl)  [unwired: 6 in, 1 out]
    n108 = feedback-in #10(w280) -> ()
    n109 = call <vilib>:"Butterworth Filter PtByPt.vi"("low cutoff freq: fl"=2.0, "sampling freq: fs"=500.0, "x"=w238) -> ("Filtered x"=w279:dbl)  [unwired: 6 in, 1 out]
    n110 = feedback-in #11(w279) -> ()
    n111 = call <vilib>:"Butterworth Filter PtByPt.vi"("low cutoff freq: fl"=2.0, "sampling freq: fs"=500.0, "x"=w236) -> ("Filtered x"=w278:dbl)  [unwired: 6 in, 1 out]
    n112 = feedback-in #12(w278) -> ()
    n113 = call "Build XY Graph"("Reset"="RESETMAP", "Y Input"=w273, "X Input"=w274) -> ("XY Graph"=→"Map":cluster{"X":dbl[], "Y":dbl[]}[])  [unwired: 7 in, 1 out]
    n114 = node-c288() -> ()  [unwired: 1 in, 1 out]
    "Real Matrix" <- w229
    "Real Matrix 2" <- w228
  }
  n115 = node-c288(w16) -> ()  [unwired: 1 out]
